vi "Write Sessions.vi"(10 "Sessions":refnum<class "Session.lvclass">[](array[class]), 11 "TCPConnectionHandler in":refnum<class "TCPConnectionHandler.lvclass">) -> (3 "TCPConnectionHandler out":refnum<class "TCPConnectionHandler.lvclass">)   [LabVIEW 2013, in "MQTT_TCP.lvlib" / "TCPConnectionHandler.lvclass"]
uses:
  TCPConnectionHandler.lvclass
  MQTT_Base/Session/Session.lvclass
  TCPConnectionHandler.lvclass/TCPConnectionHandler.ctl
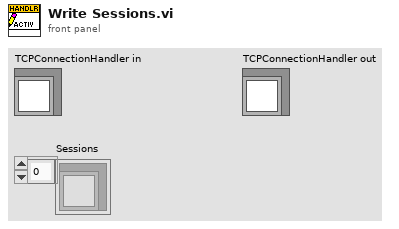
[diagram p1: front panel]
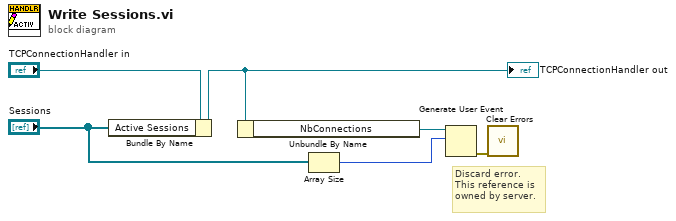
[diagram p0: block diagram]
diagram:
  # "Discard error.\nThis reference is\nowned by server."
  n1 = Bundle By Name(cluster="TCPConnectionHandler in", "Active Sessions"="Sessions") -> (w5:refnum<class "TCPConnectionHandler.lvclass">)
  "TCPConnectionHandler out" <- w5
  n2 = Unbundle By Name(w5) -> ("NbConnections"=w4:refnum<user-event>)
  n3 = Array Size(array="Sessions") -> (size(s)=w2:i32)
  n4 = Generate User Event(user event=w4, event data cluster=w2) -> (error out=w1:errorcluster)  [unwired: 2 in, 1 out]
  n5 = call <vilib>:"Clear Errors.vi"("error in (no error)"=w1) -> ()  [unwired: 6 in, 1 out]
